vi "Example All Data - AllData Callback.vi"(4 "AllData":refnum<user-event>, 5 "Event Data":T1, 6 "Control Ref":refnum<k24>, 7 "Event Common Data":T2) -> ()   [LabVIEW 2013]
uses:
  C:/tf/play/labview/Tinkerforge.dll
  Tinkerforge.dll
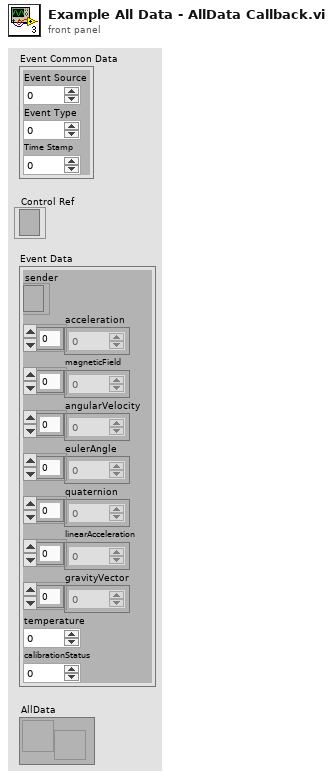
[diagram p1: front panel]
types:
  T1 = cluster{"sender":refnum<k24>, "acceleration":i16[], "magneticField":i16[], "angularVelocity":i16[], "eulerAngle":i16[], "quaternion":i16[], "linearAcceleration":i16[], "gravityVector":i16[], "temperature":i16, "calibrationStatus":u8}
  T2 = cluster{"Event Source":i32, "Event Type":u32, "Time Stamp":u32}
  T3 = cluster{"acceleration":i16[], "magneticField":i16[], "angularVelocity":i16[], "eulerAngle":i16[], "quaternion":i16[], "linearAcceleration":i16[], "gravityVector":i16[], "temperature":i16, "calibrationStatus":u8}
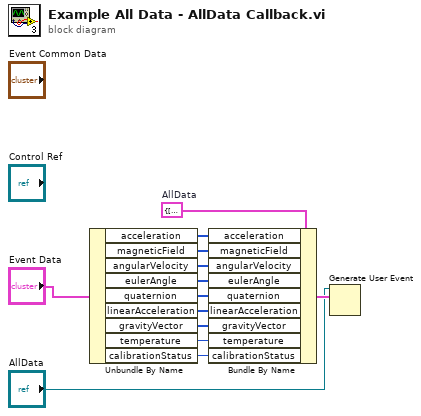
[diagram p0: block diagram]
diagram:
  w13 = T3 {"acceleration"=[], "magneticField"=[], "angularVelocity"=[], "eulerAngle"=[], "quaternion"=[], "linearAcceleration"=[], "gravityVector"=[], "temperature"=0, "calibrationStatus"=0}  # AllData
  n1 = Unbundle By Name("Event Data") -> ("acceleration"=w12:i16[], "magneticField"=w11:i16[], "angularVelocity"=w10:i16[], "eulerAngle"=w9:i16[], "quaternion"=w8:i16[], "linearAcceleration"=w7:i16[], "gravityVector"=w6:i16[], "temperature"=w5:i16, "calibrationStatus"=w4:u8)
  n2 = Bundle By Name(cluster=w13, "acceleration"=w12, "magneticField"=w11, "angularVelocity"=w10, "eulerAngle"=w9, "quaternion"=w8, "linearAcceleration"=w7, "gravityVector"=w6, "temperature"=w5, "calibrationStatus"=w4) -> (w3:T3)
  n3 = Generate User Event(user event="AllData", event data cluster=w3) -> ()  [unwired: 2 in, 2 out]
